vi "Search_and_match.vi"(0 "Learn Mode":u32(ring)=1 items=["All", "Shift Information", "Rotation Information"], 1 "Feature Mode":u32(ring) items=["Color and Shape", "Color", "Shape "], 2 "Minimum Match Score":sgl=800.0 min=0 max=1000 format="%.2f", 3 "Number of Matches Requested":i32=1 min=1, 4 "Match Mode":u32(ring) items=["Shift Invariant", "Rotation Invariant"], 6 "Ref path":path, 7 "Match Feature Mode":u32(ring)=2 items=["Color and Shape", "Color", "Shape"], 8 "Main Path":path) -> (12 "Match values":T1, 14 "Number of Matches":i32, 15 "Total Score":sgl, 16 "Shape Score":sgl, 17 "Main Image":T3(plugin-control))   [LabVIEW 2024, in "Keyence_VS150.lvlib"]
uses:
  Keyence_VS150.lvlib
  <vilib>/vision/NI_Vision_Development_Module.lvlib
panel:
  in  "Match Mode 2":u32(ring) items=["Shift Invariant", "Rotation Invariant"]
  in  "Match Feature Mode 2":u32(ring)=1 items=["Color and Shape", "Color", "Shape"]
  in  "Rotation Angle Ranges (degrees) 2":cluster{sgl, sgl}[](array[cluster]) {"?" format="%.2f"; "?" format="%.2f"}
  out "Match values 2":T1
  out "Matches 2":T2(array[cluster]) {"Bounding Box"."y" format="%.2f"; "Bounding Box"."x" format="%.2f"; "Position"."y" format="%.2f"; "Position"."x" format="%.2f"; "Score" format="%.2f"; "Scale" format="%.2f"; "Angle" format="%.2f"}
  out "error out":errorcluster
  out "Extraced_Image":T3(plugin-control)
  in  "Rotation Angle Ranges (degrees)":cluster{sgl, sgl}[](array[cluster]) {"?" format="%.2f"; "?" format="%.2f"}
  out "Ref image":T3(plugin-control)
  out "Matches":T2(array[cluster]) {"Bounding Box"."y" format="%.2f"; "Bounding Box"."x" format="%.2f"; "Position"."y" format="%.2f"; "Position"."x" format="%.2f"; "Score" format="%.2f"; "Scale" format="%.2f"; "Angle" format="%.2f"}
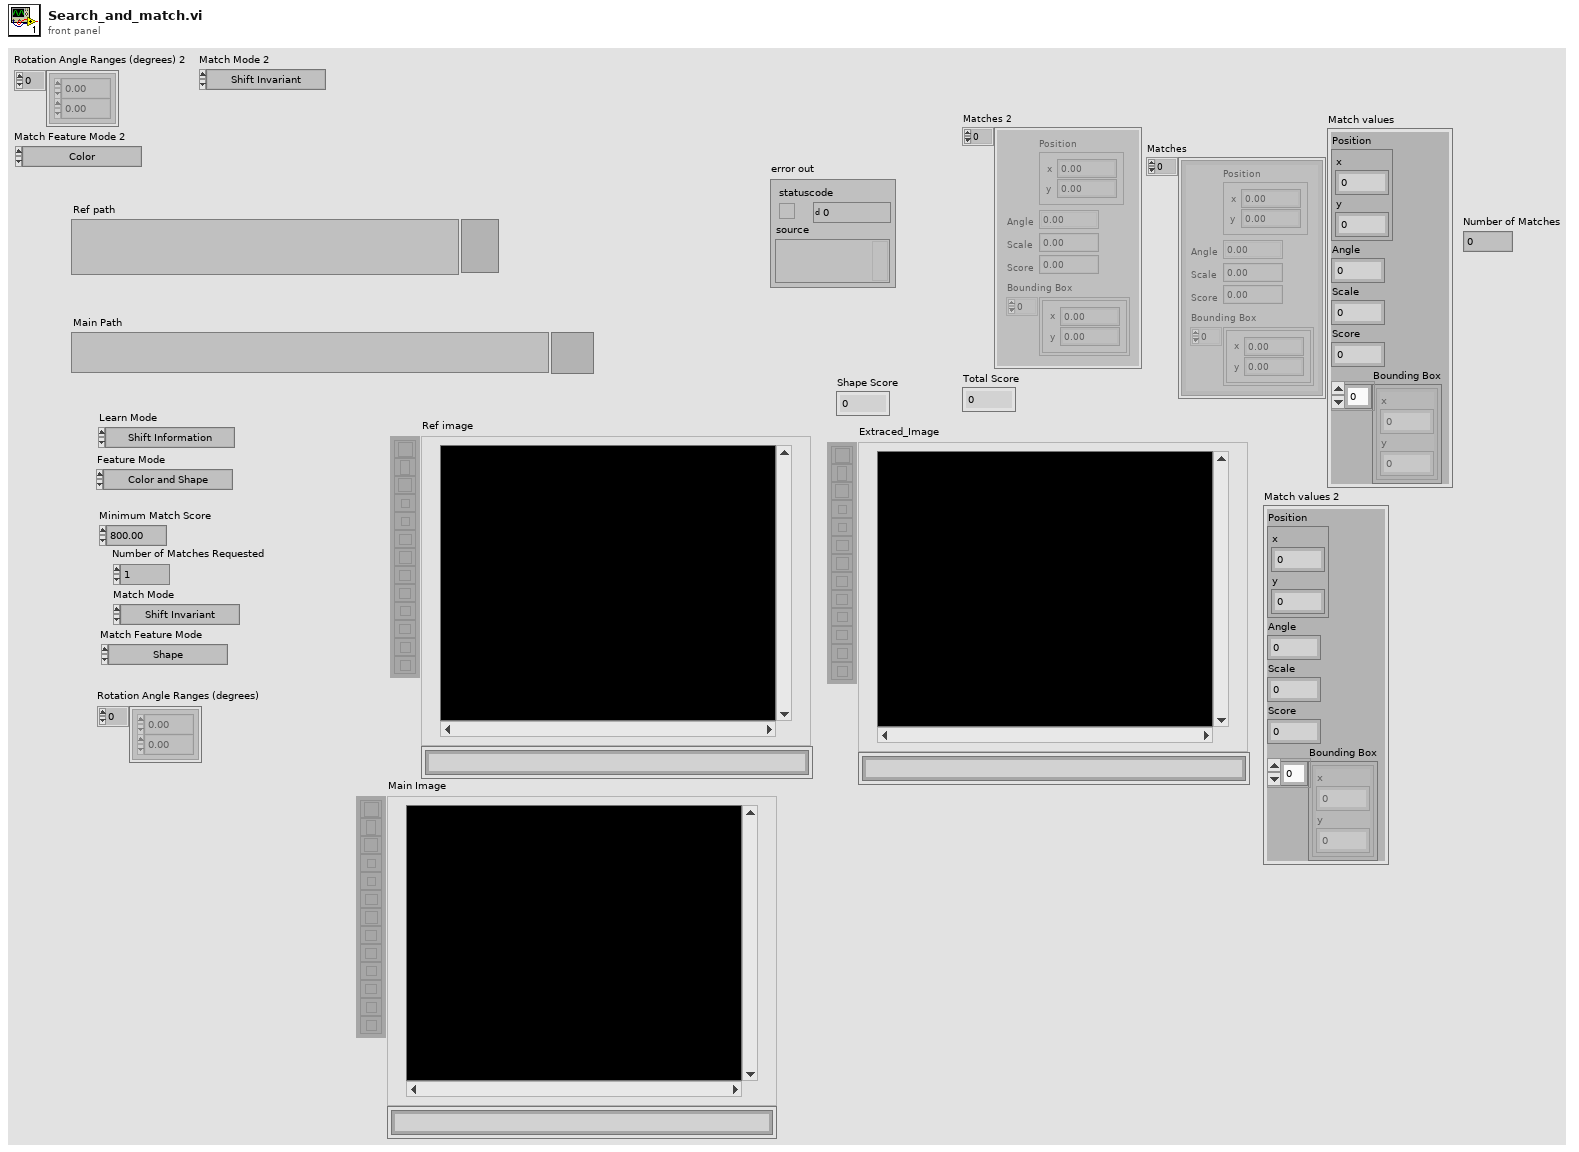
[diagram p1: front panel]
types:
  T1 = cluster{"Position":cluster{"x":sgl, "y":sgl}, "Angle":sgl, "Scale":sgl, "Score":sgl, "Bounding Box":cluster{"x":sgl, "y":sgl}[]}
  T2 = cluster{"Position":cluster{"x":sgl, "y":sgl}, "Angle":sgl, "Scale":sgl, "Score":sgl, "Bounding Box":cluster{"x":sgl, "y":sgl}[]}[]
  T3 = typedef "IMAQ Image.ctl" = refnum<image>
  T4 = typedef "Image Type" = u32
  T5 = typedef "IMAQ Rectangle" = cluster{"Left":i32, "Top":i32, "Right":i32, "Bottom":i32, "Rotation":dbl}
  T6 = typedef "ROI Descriptor" = cluster{"Global Rectangle":i32[], "Contours":cluster{"ID":enum32{"External", "Internal"}, "Type":u32, "Coordinates":i32[]}[]}
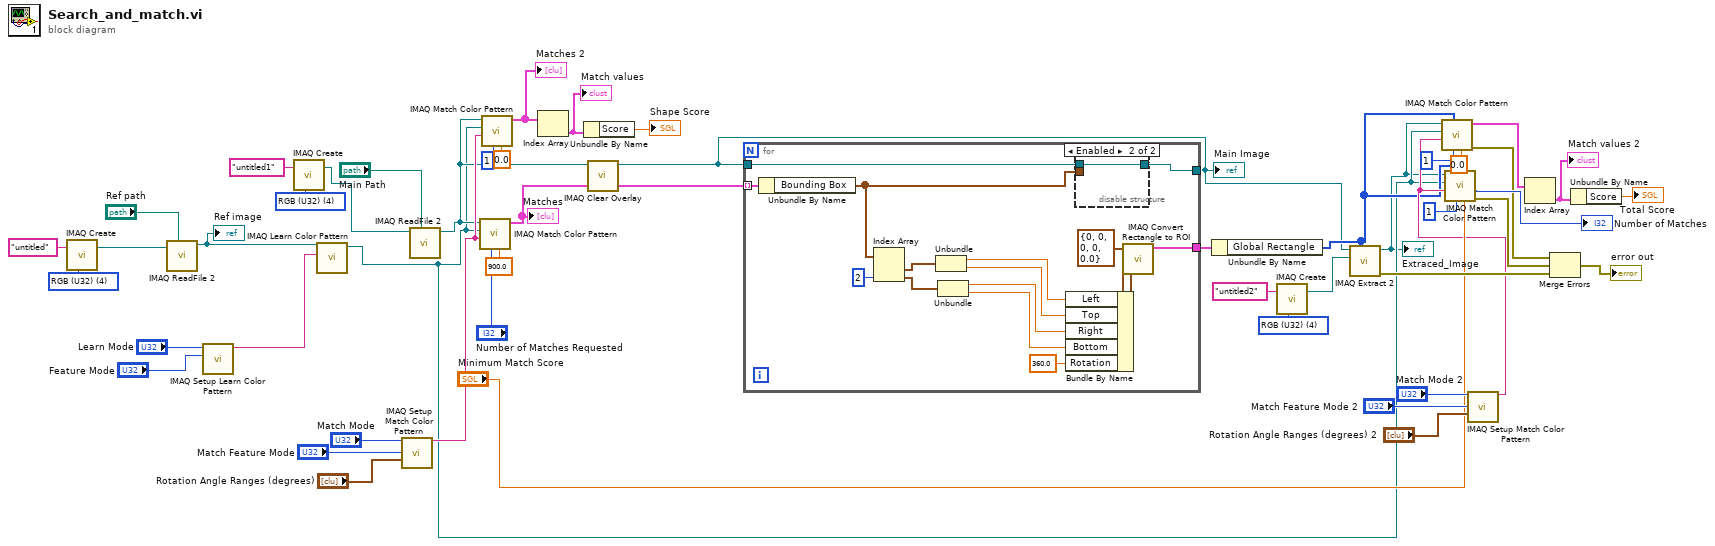
[diagram p0: block diagram]
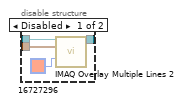
[diagram p2: hidden frame]
diagram:
  w34 = T4 4 items=["Grayscale (U8)", "Grayscale (I16)", "Grayscale (SGL)", "Complex (CSG)", "RGB (U32)", "HSL (U32)", "RGB (U64)", "Grayscale (U16)"] ("Image Type")
  w45 = T4 4 items=["Grayscale (U8)", "Grayscale (I16)", "Grayscale (SGL)", "Complex (CSG)", "RGB (U32)", "HSL (U32)", "RGB (U64)", "Grayscale (U16)"] ("Image Type")
  w48 = T4 4 items=["Grayscale (U8)", "Grayscale (I16)", "Grayscale (SGL)", "Complex (CSG)", "RGB (U32)", "HSL (U32)", "RGB (U64)", "Grayscale (U16)"] ("Image Type")
  n1 = call "IMAQ Create"("Image Name"="untitled", "Image Type"=w48) -> ("New Image"=w47:T3)  [unwired: 3 in, 1 out]
  n2 = call "IMAQ ReadFile 2"("File Path"="Ref path", "Image"=w47) -> ("Image Out"=w36:T3)  [unwired: 5 in, 4 out]
  "Ref image" <- w36
  n3 = call "IMAQ Setup Learn Color Pattern"("Feature Mode"="Feature Mode", "Learn Mode"="Learn Mode") -> ("Learn Color Pattern Setup Data"=w41:string)  [unwired: 8 in, 1 out]
  n4 = call "IMAQ Create"("Image Name"="untitled1", "Image Type"=w45) -> ("New Image"=w40:T3)  [unwired: 3 in, 1 out]
  n5 = call "IMAQ Learn Color Pattern"("Learn Color Pattern Setup Data"=w41, "Image"=w36) -> ("Template Image Out"=w2:T3)  [unwired: 8 in, 1 out]
  n6 = call "IMAQ Setup Match Color Pattern"("Match Mode"="Match Mode", "Match Feature Mode"="Match Feature Mode", "Rotation Angle Ranges (degrees)"="Rotation Angle Ranges (degrees)") -> ("Match Color Pattern Setup Data"=w30:string)  [unwired: 11 in, 1 out]
  n7 = call "IMAQ ReadFile 2"("File Path"="Main Path", "Image"=w40) -> ("Image Out"=w8:T3)  [unwired: 5 in, 4 out]
  n8 = call "IMAQ Match Color Pattern"("Minimum Match Score"=sgl 900.0, "Number of Matches Requested"="Number of Matches Requested", "Match Color Pattern Setup Data"=w30, "Template Image"=w2, "Image"=w8) -> ("Matches"=w20:T2)  [unwired: 4 in, 2 out]
  "Matches" <- w20
  n9 = call "IMAQ Match Color Pattern"("Minimum Match Score"=sgl 0.0, "Number of Matches Requested"=1, "Match Color Pattern Setup Data"=w30, "Template Image"=w2, "Image"=w8) -> ("Matches"=w27:T2)  [unwired: 4 in, 2 out]
  "Matches 2" <- w27
  n10 = Index Array(array=w27) -> (element=w26:T1)  [unwired: 1 in]
  "Match values" <- w26
  n11 = Unbundle By Name(w26) -> ("Score"=→"Shape Score":sgl)
  n12 = call "IMAQ Clear Overlay"("Image"=w8) -> ("Image Out"=w4:T3)  [unwired: 9 in, 1 out]
  "Main Image" <- w4
  n13 = for {
    tunnel: w4 -> [w64]
    tunnel: w20 -> [w63] mode=indexing
    tunnel: [w62] -> _
    tunnel: [w51] -> w3
    n14 = Unbundle By Name(w63) -> ("Bounding Box"=w58:cluster{"x":sgl, "y":sgl}[])
    n15 = Index Array(array=w58, index #2=2 ("index")) -> (element #1=w57:cluster{"x":sgl, "y":sgl}, element #2=w56:cluster{"x":sgl, "y":sgl})  [unwired: 1 in]
    n16 = Unbundle(w57) -> ("x"=w55:sgl, "y"=w54:sgl)
    n17 = Unbundle(w56) -> ("x"=w53:sgl, "y"=w52:sgl)
    n18 = Bundle By Name(cluster=T5 {"Left"=0, "Top"=0, "Right"=0, "Bottom"=0, "Rotation"=0.0} ("Rectangle"), "Left"=w55, "Top"=w54, "Right"=w53, "Bottom"=w52, "Rotation"=360.0) -> (w60:T5)
    n19 = disable-structure shown="Enabled" {
      disable-tunnel: w64 -> [w68 w69]
      disable-tunnel: [w66 w69] -> w62
      disable-tunnel: w58 -> [w65 _]
      frame Disabled {
        n20 = call "IMAQ Overlay Multiple Lines 2"("Image"=w68, "Line End Points"=w65, "Color"=u32 16727296) -> ("Image Out"=w66:T3)  [unwired: 11 in, 1 out]
      }
      frame Enabled {
      }
    }
    n21 = call "IMAQ Convert Rectangle to ROI"("Rectangle"=w60) -> ("ROI Descriptor"=w51:T6)  [unwired: 8 in, 1 out]
  }
  n22 = Unbundle By Name(w3) -> ("Global Rectangle"=w5:i32[])
  n23 = call "IMAQ Create"("Image Name"="untitled2", "Image Type"=w34) -> ("New Image"=w32:T3)  [unwired: 3 in, 1 out]
  n24 = call "IMAQ Extract 2"("Optional Rectangle"=w5, "Image Dst"=w32, "Image Src"=w4) -> ("error out"=w31:errorcluster, "Image Dst Out"=w1:T3)  [unwired: 7 in]
  "Extraced_Image" <- w1
  n25 = call "IMAQ Setup Match Color Pattern"("Match Mode"="Match Mode 2", "Match Feature Mode"="Match Feature Mode 2", "Rotation Angle Ranges (degrees)"="Rotation Angle Ranges (degrees) 2") -> ("Match Color Pattern Setup Data"=w13:string)  [unwired: 11 in, 1 out]
  n26 = call "IMAQ Match Color Pattern"("Minimum Match Score"=sgl 0.0, "Number of Matches Requested"=1, "Optional Rectangle"=w5, "Match Color Pattern Setup Data"=w13, "Template Image"=w2, "Image"=w1) -> ("error out"=w9:errorcluster, "Matches"=w10:T2)  [unwired: 3 in, 1 out]
  n27 = call "IMAQ Match Color Pattern"("Minimum Match Score"="Minimum Match Score", "Number of Matches Requested"=1, "Optional Rectangle"=w5, "Match Color Pattern Setup Data"=w13, "Template Image"=w2, "Image"=w1) -> ("error out"=w18:errorcluster, "Number of Matches"=→"Number of Matches":i32)  [unwired: 3 in, 1 out]
  n28 = Index Array(array=w10) -> (element=w24:T1)  [unwired: 1 in]
  "Match values 2" <- w24
  n29 = Merge Errors(w9, w18, w31) -> (→"error out":errorcluster)
  n30 = Unbundle By Name(w24) -> ("Score"=→"Total Score":sgl)
